vi "PCO_RecorderSaveImage_B8.vi"(0 "pImgBuf":u8[][](array[numeric])=array1x4097[4097 elements], 1 "wWidth":u16, 2 "wHeight":u16, 3 "szFilePath":path, 5 "error in (no error)":errorcluster {"code" format="%x"}, 6 "isColor":bool, 8 "bIsBitmap":bool, 9 "PCO_METADATA_STRUCT":T1={"wVersion"=65535, "dwIMAGE_COUNTER"=0, "dwIMAGE_TIME_US"=0, "lvTimestamp"=timestamp(0 s since 1904-01-01), "bIMAGE_TIME_STATUS"=0, "wEXPOSURE_TIME_BASE"=0, "dwEXPOSURE_TIME"=0, "dwFRAMERATE_MILLIHZ"=0, "sSENSOR_TEMPERATURE"=0, "wIMAGE_SIZE_X"=0, "wIMAGE_SIZE_Y"=0, "bBINNING_X"=0, "bBINNING_Y"=0, "dwSENSOR_READOUT_FREQUENCY"=0, "wSENSOR_CONV_FACTOR"=0, "dwCAMERA_SERIAL_NO"=0, "wCAMERA_TYPE"=0, "bBIT_RESOLUTION"=0, "bSYNC_STATUS"=0, "wDARK_OFFSET"=0, "bTRIGGER_MODE"=0, "bDOUBLE_IMAGE_MODE"=0, "bCAMERA_SYNC_MODE"=0, "bIMAGE_TYPE"=0, "wCOLOR_PATTERN"=0, "wCAMERA_SUBTYPE"=0, "dwEVENT_NUMBER"=0, "wIMAGE_SIZE_X_Offset"=0, "wIMAGE_SIZE_Y_Offset"=0}, 10 "bOverwrite":bool) -> (14 "ErrorMessage":i32 format="%x", 19 "error out":errorcluster {"code" format="%x"})   [LabVIEW 2020, in "Recorder.lvlib"]
doc: "int WINAPI PCO_RecorderSaveImage(void* pImgBuf, WORD wWidth, WORD wHeight, const char* cFileType, bool bIsBitmap, const char* szFilePath, bool bOverwrite, PCO_METADATA_STRUCT* strMetadata);"
uses:
  Recorder.lvlib
  Structures.lvlib
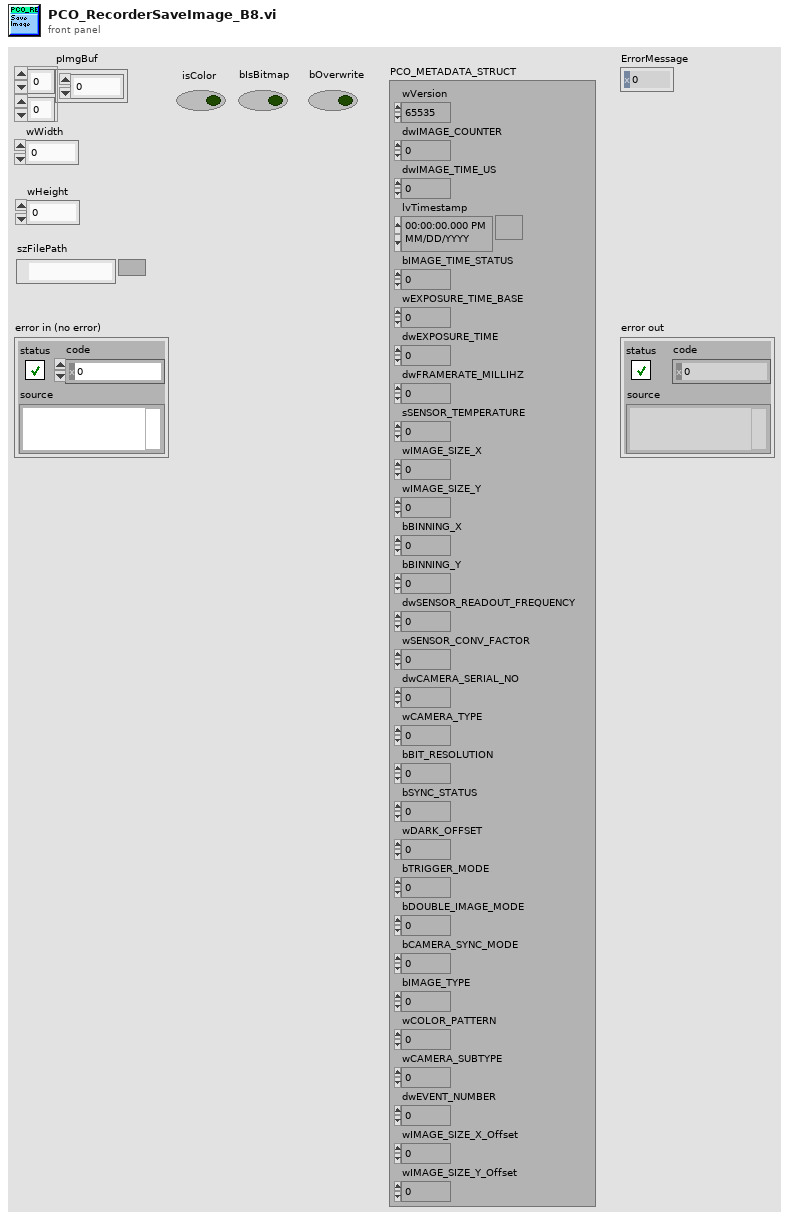
[diagram p1: front panel]
types:
  T1 = cluster{"wVersion":u16, "dwIMAGE_COUNTER":u32, "dwIMAGE_TIME_US":u32, "lvTimestamp":timestamp, "bIMAGE_TIME_STATUS":u8, "wEXPOSURE_TIME_BASE":u16, "dwEXPOSURE_TIME":u32, "dwFRAMERATE_MILLIHZ":u32, "sSENSOR_TEMPERATURE":i16, "wIMAGE_SIZE_X":u16, "wIMAGE_SIZE_Y":u16, "bBINNING_X":u8, "bBINNING_Y":u8, "dwSENSOR_READOUT_FREQUENCY":u32, "wSENSOR_CONV_FACTOR":u16, "dwCAMERA_SERIAL_NO":u32, "wCAMERA_TYPE":u16, "bBIT_RESOLUTION":u8, "bSYNC_STATUS":u8, "wDARK_OFFSET":u16, "bTRIGGER_MODE":u8, "bDOUBLE_IMAGE_MODE":u8, "bCAMERA_SYNC_MODE":u8, "bIMAGE_TYPE":u8, "wCOLOR_PATTERN":u16, "wCAMERA_SUBTYPE":u16, "dwEVENT_NUMBER":u32, "wIMAGE_SIZE_X_Offset":u16, "wIMAGE_SIZE_Y_Offset":u16}
  T2 = typedef "LVDateTimeRec.ctl" = cluster{"fractional second":dbl, "second":i32, "minute":i32, "hour":i32, "day of month":i32, "month":i32, "year":i32, "day of week":i32, "day of year":i32, "DST":i32}
  T3 = cluster{"wSize":u16, "wVersion":u16, "bIMAGE_COUNTER_BCD":cluster{u8, u8, u8, u8}, "bIMAGE_TIME_US_BCD":cluster{u8, u8, u8}, "bIMAGE_TIME_SEC_BCD":u8, "bIMAGE_TIME_MIN_BCD":u8, "bIMAGE_TIME_HOUR_BCD":u8, "bIMAGE_TIME_DAY_BCD":u8, "bIMAGE_TIME_MON_BCD":u8, "bIMAGE_TIME_YEAR_BCD":u8, "bIMAGE_TIME_STATUS":u8, "wEXPOSURE_TIME_BASE":u16, "dwEXPOSURE_TIME":u32, "dwFRAMERATE_MILLIHZ":u32, "sSENSOR_TEMPERATURE":i16, "wIMAGE_SIZE_X":u16, "wIMAGE_SIZE_Y":u16, "bBINNING_X":u8, "bBINNING_Y":u8, "dwSENSOR_READOUT_FREQUENCY":u32, "wSENSOR_CONV_FACTOR":u16, "dwCAMERA_SERIAL_NO":u32, "wCAMERA_TYPE":u16, "bBIT_RESOLUTION":u8, "bSYNC_STATUS":u8, "wDARK_OFFSET":u16, "bTRIGGER_MODE":u8, "bDOUBLE_IMAGE_MODE":u8, "bCAMERA_SYNC_MODE":u8, "bIMAGE_TYPE":u8, "wCOLOR_PATTERN":u16, "wCAMERA_SUBTYPE":u16, "dwEVENT_NUMBER":u32, "wIMAGE_SIZE_X_Offset":u16, "wIMAGE_SIZE_Y_Offset":u16}
  T4 = enum16{"big-endian, network order", "native, host order", "little-endian"}
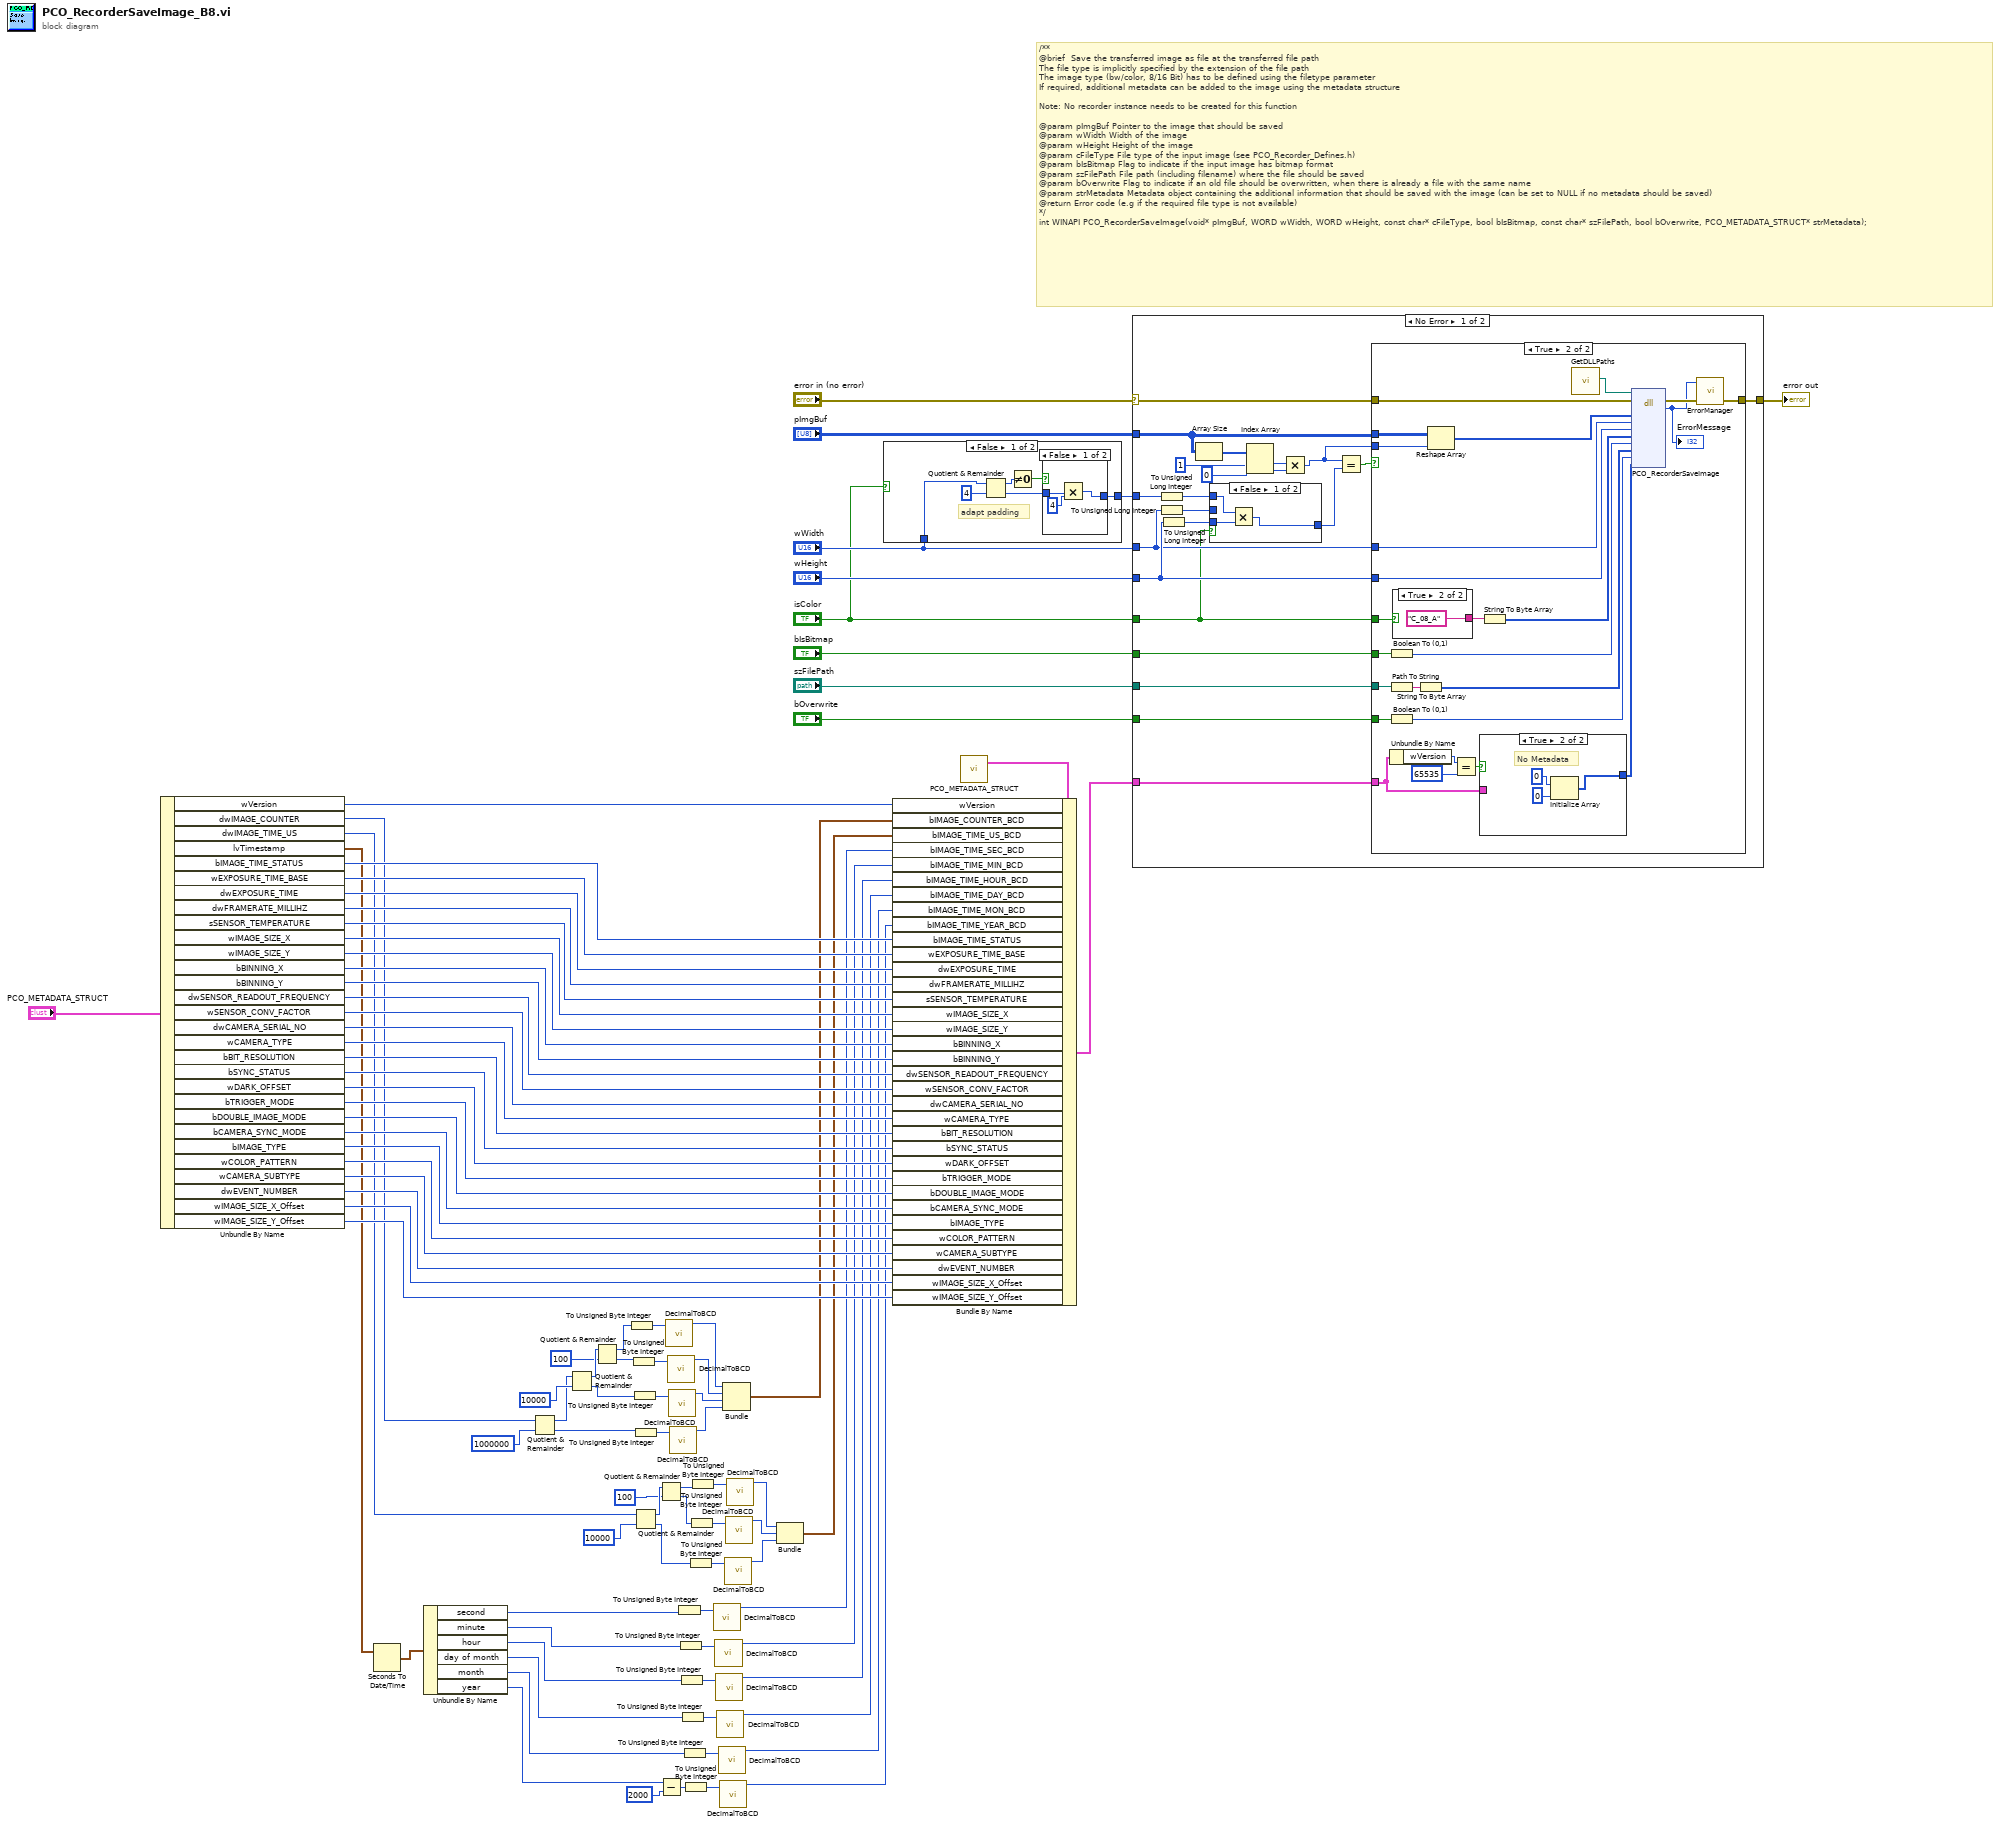
[diagram p0: block diagram]
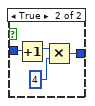
[diagram p2: hidden frame]
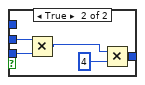
[diagram p4: hidden frame]
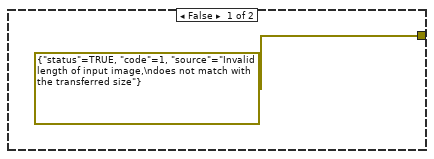
[diagram p5: hidden frame]
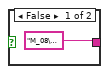
[diagram p6: hidden frame]
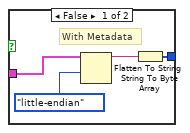
[diagram p7: hidden frame]
diagram:
  # "/**\n@brief  Save the transferred image as file at the transferred file path\nThe file type is implicitly specified by the extension of the file path\nThe image type (bw/color, 8/16 Bit) has to be defined using the filetype parameter\nIf required, additional metadata can be added to the image using the metadata structure\n\nNote: No recorder instance needs to be created for this function\n\n@param pImgBuf Pointer to the image that should be saved\n@param wWidth Width of the image\n@param wHeight Height of the image\n@param cFileType File type of the input image (see PCO_Recorder_Defines.h)\n@param bIsBitmap Flag to indicate if the input image has bitmap format\n@param szFilePath File path (including filename) where the file should be saved\n@param bOverwrite Flag to indicate if an old file should be overwritten, when there is already a file with the same name\n@param strMetadata Metadata object containing the additional information that should be saved with the image (can be set to NULL if no metadata should be saved)\n@return Error code (e.g if the required file type is not available)\n*/\nint WINAPI PCO_RecorderSaveImage(void* pImgBuf, WORD wWidth, WORD wHeight, const char* cFileType, bool bIsBitmap, const char* szFilePath, bool bOverwrite, PCO_METADATA_STRUCT* strMetadata);"
  n1 = Unbundle By Name("PCO_METADATA_STRUCT") -> ("wVersion"=w82:u16, "dwIMAGE_COUNTER"=w16:u32, "dwIMAGE_TIME_US"=w21:u32, "lvTimestamp"=w56:timestamp, "bIMAGE_TIME_STATUS"=w70:u8, "wEXPOSURE_TIME_BASE"=w57:u16, "dwEXPOSURE_TIME"=w58:u32, "dwFRAMERATE_MILLIHZ"=w59:u32, "sSENSOR_TEMPERATURE"=w60:i16, "wIMAGE_SIZE_X"=w61:u16, "wIMAGE_SIZE_Y"=w62:u16, "bBINNING_X"=w63:u8, "bBINNING_Y"=w64:u8, "dwSENSOR_READOUT_FREQUENCY"=w65:u32, "wSENSOR_CONV_FACTOR"=w66:u16, "dwCAMERA_SERIAL_NO"=w67:u32, "wCAMERA_TYPE"=w68:u16, "bBIT_RESOLUTION"=w69:u8, "bSYNC_STATUS"=w71:u8, "wDARK_OFFSET"=w72:u16, "bTRIGGER_MODE"=w73:u8, "bDOUBLE_IMAGE_MODE"=w74:u8, "bCAMERA_SYNC_MODE"=w75:u8, "bIMAGE_TYPE"=w76:u8, "wCOLOR_PATTERN"=w77:u16, "wCAMERA_SUBTYPE"=w78:u16, "dwEVENT_NUMBER"=w79:u32, "wIMAGE_SIZE_X_Offset"=w80:u16, "wIMAGE_SIZE_Y_Offset"=w81:u16)
  n2 = Seconds To Date/Time(time stamp (now)=w56) -> (date time rec=w55:T2)  [unwired: 1 in]
  n3 = Unbundle By Name(w55) -> ("second"=w54:i32, "minute"=w51:i32, "hour"=w46:i32, "day of month"=w45:i32, "month"=w44:i32, "year"=w41:i32)
  n4 = Quotient & Remainder(x=w16, y=u32 1000000 ("x")) -> (x-y*floor(x/y)=w15:u32, floor(x/y)=w10:u32)
  n5 = Quotient & Remainder(x=w15, y=u32 10000 ("x")) -> (x-y*floor(x/y)=w19:u32, floor(x/y)=w9:u32)
  n6 = Quotient & Remainder(x=w19, y=u32 100 ("x")) -> (x-y*floor(x/y)=w7:u32, floor(x/y)=w8:u32)
  n7 = To Unsigned Byte Integer(number=w7) -> (unsigned 8bit integer=w14:u8)
  n8 = To Unsigned Byte Integer(number=w8) -> (unsigned 8bit integer=w13:u8)
  n9 = To Unsigned Byte Integer(number=w9) -> (unsigned 8bit integer=w12:u8)
  n10 = To Unsigned Byte Integer(number=w10) -> (unsigned 8bit integer=w11:u8)
  n11 = Quotient & Remainder(x=w21, y=u32 10000 ("x")) -> (x-y*floor(x/y)=w33:u32, floor(x/y)=w26:u32)
  n12 = Quotient & Remainder(x=w33, y=u32 100 ("x")) -> (x-y*floor(x/y)=w30:u32, floor(x/y)=w28:u32)
  n13 = Subtract(x=w41, y=2000) -> (x-y=w42:i32)
  n14 = call "DecimalToBCD.vi"("U8"=w14) -> ("BCD"=w6:u8)  [unwired: 10 in]
  n15 = call "DecimalToBCD.vi"("U8"=w13) -> ("BCD"=w5:u8)  [unwired: 10 in]
  n16 = call "DecimalToBCD.vi"("U8"=w12) -> ("BCD"=w4:u8)  [unwired: 10 in]
  n17 = call "DecimalToBCD.vi"("U8"=w11) -> ("BCD"=w3:u8)  [unwired: 10 in]
  n18 = To Unsigned Byte Integer(number=w54) -> (unsigned 8bit integer=w53:u8)
  n19 = To Unsigned Byte Integer(number=w51) -> (unsigned 8bit integer=w52:u8)
  n20 = To Unsigned Byte Integer(number=w46) -> (unsigned 8bit integer=w50:u8)
  n21 = To Unsigned Byte Integer(number=w45) -> (unsigned 8bit integer=w47:u8)
  n22 = To Unsigned Byte Integer(number=w44) -> (unsigned 8bit integer=w48:u8)
  n23 = To Unsigned Byte Integer(number=w42) -> (unsigned 8bit integer=w49:u8)
  n24 = To Unsigned Byte Integer(number=w26) -> (unsigned 8bit integer=w27:u8)
  n25 = To Unsigned Byte Integer(number=w28) -> (unsigned 8bit integer=w29:u8)
  n26 = To Unsigned Byte Integer(number=w30) -> (unsigned 8bit integer=w31:u8)
  n27 = call "DecimalToBCD.vi"("U8"=w53) -> ("BCD"=w35:u8)  [unwired: 10 in]
  n28 = call "DecimalToBCD.vi"("U8"=w52) -> ("BCD"=w36:u8)  [unwired: 10 in]
  n29 = call "DecimalToBCD.vi"("U8"=w50) -> ("BCD"=w37:u8)  [unwired: 10 in]
  n30 = call "DecimalToBCD.vi"("U8"=w47) -> ("BCD"=w38:u8)  [unwired: 10 in]
  n31 = call "DecimalToBCD.vi"("U8"=w48) -> ("BCD"=w39:u8)  [unwired: 10 in]
  n32 = call "DecimalToBCD.vi"("U8"=w49) -> ("BCD"=w40:u8)  [unwired: 10 in]
  n33 = Bundle("BCD"=w6, "BCD"=w5, "BCD"=w4, "BCD"=w3) -> (w2:cluster{"BCD":u8, "BCD":u8, "BCD":u8, "BCD":u8})  [unwired: 1 in]
  n34 = call "DecimalToBCD.vi"("U8"=w27) -> ("BCD"=w23:u8)  [unwired: 10 in]
  n35 = call "DecimalToBCD.vi"("U8"=w29) -> ("BCD"=w24:u8)  [unwired: 10 in]
  n36 = call "DecimalToBCD.vi"("U8"=w31) -> ("BCD"=w25:u8)  [unwired: 10 in]
  n37 = Bundle("BCD"=w25, "BCD"=w24, "BCD"=w23) -> (w22:cluster{"BCD":u8, "BCD":u8, "BCD":u8})  [unwired: 1 in]
  n38 = case shown="False" "isColor" {
    tunnel: "wWidth" -> [w96 w108]
    tunnel: [w95 w108] -> w86
    frame False {
      # "adapt padding"
      n39 = Quotient & Remainder(x=w96, y=u16 4) -> (x-y*floor(x/y)=w99:u16, floor(x/y)=w97:u16)
      n40 = Not Equal To 0?(x=w99) -> (x != 0?=w98:bool)
      n41 = case shown="False" w98 {
        tunnel: w97 -> [w103 w107]
        tunnel: [w101 w104] -> w95
        frame False {
          n42 = Multiply(x=w103, y=u16 4) -> (x*y=w101:u16)
        }
        frame True {
          n43 = Increment(x=w107) -> (x+1=w105:u16)
          n44 = Multiply(x=w105, y=u16 4) -> (x*y=w104:u16)
        }
      }
    }
    frame True {
    }
  }
  n45 = call "PCO_METADATA_STRUCT.vi"() -> ("PCO_METADATA_STRUCT_Raw"=w84:T3)  [unwired: 4 in, 3 out]
  n46 = Bundle By Name(cluster=w84, "wVersion"=w82, "bIMAGE_COUNTER_BCD"=w2, "bIMAGE_TIME_US_BCD"=w22, "bIMAGE_TIME_SEC_BCD"=w35, "bIMAGE_TIME_MIN_BCD"=w36, "bIMAGE_TIME_HOUR_BCD"=w37, "bIMAGE_TIME_DAY_BCD"=w38, "bIMAGE_TIME_MON_BCD"=w39, "bIMAGE_TIME_YEAR_BCD"=w40, "bIMAGE_TIME_STATUS"=w70, "wEXPOSURE_TIME_BASE"=w57, "dwEXPOSURE_TIME"=w58, "dwFRAMERATE_MILLIHZ"=w59, "sSENSOR_TEMPERATURE"=w60, "wIMAGE_SIZE_X"=w61, "wIMAGE_SIZE_Y"=w62, "bBINNING_X"=w63, "bBINNING_Y"=w64, "dwSENSOR_READOUT_FREQUENCY"=w65, "wSENSOR_CONV_FACTOR"=w66, "dwCAMERA_SERIAL_NO"=w67, "wCAMERA_TYPE"=w68, "bBIT_RESOLUTION"=w69, "bSYNC_STATUS"=w71, "wDARK_OFFSET"=w72, "bTRIGGER_MODE"=w73, "bDOUBLE_IMAGE_MODE"=w74, "bCAMERA_SYNC_MODE"=w75, "bIMAGE_TYPE"=w76, "wCOLOR_PATTERN"=w77, "wCAMERA_SUBTYPE"=w78, "dwEVENT_NUMBER"=w79, "wIMAGE_SIZE_X_Offset"=w80, "wIMAGE_SIZE_Y_Offset"=w81) -> (w83:T3)
  n47 = case shown="No Error" "error in (no error)" {
    selector: "error in (no error)" -> [w129 w174]
    tunnel: "pImgBuf" -> [w128 _]
    tunnel: "wWidth" -> [w115 _]
    tunnel: "wHeight" -> [w116 _]
    tunnel: "bIsBitmap" -> [w122 _]
    tunnel: [w130 w174] -> w91
    tunnel: "szFilePath" -> [w123 _]
    tunnel: "bOverwrite" -> [w124 _]
    tunnel: "isColor" -> [w110 _]
    tunnel: w83 -> [w125 _]
    tunnel: w86 -> [w114 _]
    frame No Error {
      n48 = To Unsigned Long Integer(number=w114) -> (unsigned 32bit integer=w113:u32)
      n49 = To Unsigned Long Integer(number=w115) -> (unsigned 32bit integer=w112:u32)
      n50 = To Unsigned Long Integer(number=w116) -> (unsigned 32bit integer=w111:u32)
      n51 = Array Size(array=w128) -> (size(s)=w121:i32[])
      n52 = case shown="False" w110 {
        tunnel: [w131 w137] -> w127
        tunnel: w113 -> [w132 _]
        tunnel: w112 -> [_ w135]
        tunnel: w111 -> [w133 w136]
        frame False {
          n53 = Multiply(x=w132, y=w133) -> (x*y=w131:u32)
        }
        frame True {
          n54 = Multiply(x=w135, y=w136) -> (x*y=w134:u32)
          n55 = Multiply(x=w134, y=u32 4) -> (x*y=w137:u32)
        }
      }
      n56 = Index Array(array=w121, index #1=u32 0 ("index"), index #2=u32 1 ("index")) -> (element #1=w117:i32, element #2=w118:i32)
      n57 = Multiply(x=w117, y=w118) -> (x*y=w109:u32)
      n58 = Equal?(x=w109, y=w127) -> (x = y?=w126:bool)
      n59 = case shown="True" w126 {
        tunnel: w128 -> [_ w142]
        tunnel: w115 -> [_ w164]
        tunnel: w116 -> [_ w163]
        tunnel: w122 -> [_ w162]
        tunnel: [errorcluster {"status"=TRUE, "code"=1, "source"="Invalid length of input image,\ndoes not match with the transferred size"} ("error out") w156] -> w130
        tunnel: w129 -> [_ w159]
        tunnel: w110 -> [_ w148]
        tunnel: w125 -> [_ w150]
        tunnel: w124 -> [_ w149]
        tunnel: w123 -> [_ w146]
        tunnel: w109 -> [_ w140]
        frame False {
        }
        frame True {
          n60 = Boolean To (0,1)(Boolean=w162) -> (0, 1=w161:i16)
          n61 = Path To String(path=w146) -> (string=w147:string)
          n62 = Boolean To (0,1)(Boolean=w149) -> (0, 1=w160:i16)
          n63 = Unbundle By Name(w150) -> ("wVersion"=w154:u16)
          n64 = case shown="True" w148 {
            tunnel: ["M_08\u0000" "C_08_A"] -> w144
            frame False {
            }
            frame True {
            }
          }
          n65 = String To Byte Array(string=w147) -> (unsigned byte array=w145:u8[])
          n66 = Reshape Array(w142, w140) -> (w141:u8[])
          n67 = Equal?(x=w154, y=u16 65535) -> (x = y?=w152:bool)
          n68 = case shown="True" w152 {
            tunnel: [w168 w171] -> w151
            tunnel: w150 -> [w169 _]
            frame False {
              # "With Metadata"
              n69 = Flatten To String(anything=w169, byte order (0:big-endian, network order)=T4."little-endian" ("Byte-Reihenfolge (0:Big-Endian, Netzwerkreihenfolge)")) -> (data string=w170:string)  [unwired: 2 in, 2 out]
              n70 = String To Byte Array(string=w170) -> (unsigned byte array=w168:u8[])
            }
            frame True {
              # "No Metadata"
              n71 = Initialize Array(u8 0, 0 ("dimension size")) -> (w171:u8[])
            }
          }
          n72 = String To Byte Array(string=w144) -> (unsigned byte array=w143:u8[])
          n73 = call "GetDLLPaths.vi"() -> ("PCO_Recorder_Path"=w158:path)  [unwired: 9 in, 2 out]
          n74 = dll-call lib="?" fn="PCO_RecorderSaveImage"(path in=w158, error in=w159, "pImgBuf"=w141, "wWidth"=w164, "wHeight"=w163, "cFileType"=w143, "bIsBitmap"=w161, "szFilePath"=w145, "bOverwrite"=w160, "strMetadata"=w151) -> (error out=w157:errorcluster, "return type"=w155:i32)  [unwired: 9 in, 1 out]
          "ErrorMessage" <- w155
          n75 = call "ErrorManager.vi"("error in (no error)"=w157, "error code"=w155) -> ("error out"=w156:errorcluster)  [unwired: 3 in]
        }
      }
    }
    frame Error {
    }
  }
  "error out" <- w91
